vi "Sender UI.vi"(11 "error in (no error)":errorcluster) -> (15 "error out":errorcluster)   [LabVIEW 2023, in "Sender.lvclass"]
uses:
  Sender.lvclass
  Controls/Communication Mode.ctl
  Controls/Operation.ctl
  Controls/State Cluster.ctl
  Controls/Sender Data Cluster.ctl
  Communication/Communication.lvclass
  Controls/User Event Operation.ctl
  Downloads/Sample PC Template/Sample PC Template/Typedefs/Data.ctl
  Sender.lvclass/Sender.ctl
  Downloads/Sample PC Template/Sample PC Template/Sample PC Template.lvlib
panel:
  in  "Stop Data":bool
  in  "Transmission Type":T1
  in  "Data Type":string(combo)
  in  "Send":bool
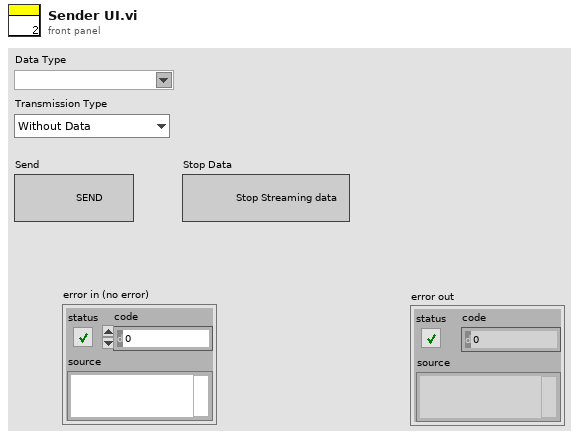
[diagram p1: front panel]
types:
  T1 = typedef "Communication Mode.ctl" = enum16{"Without Data", "With Data", "Stream Data"}
  T2 = typedef "User Event Operation.ctl" = enum16{"Obtain", "Generate", "Release"}
  T3 = typedef "Sender Data Cluster.ctl" = cluster{"user event out":refnum<user-event>, "Selected Data Type":string, "Receiver VI Reference":refnum<vi>, "Transmission Type":T1, "Start Time":dbl, "Stop Stream Data":bool, "Parent class object":refnum<class "Communication.lvclass">}
  T4 = typedef "State Cluster.ctl" = cluster{"State":string, "Data":variant}
  T5 = typedef "Operation.ctl" = enum16{"Create", "Enqueue", "Enqueue N", "Enstack", "Dequeue", "Flush", "Release"}
  T6 = typedef "Sample PC Template.lvlib/Data.ctl" = cluster{"State":string, "Data":variant}
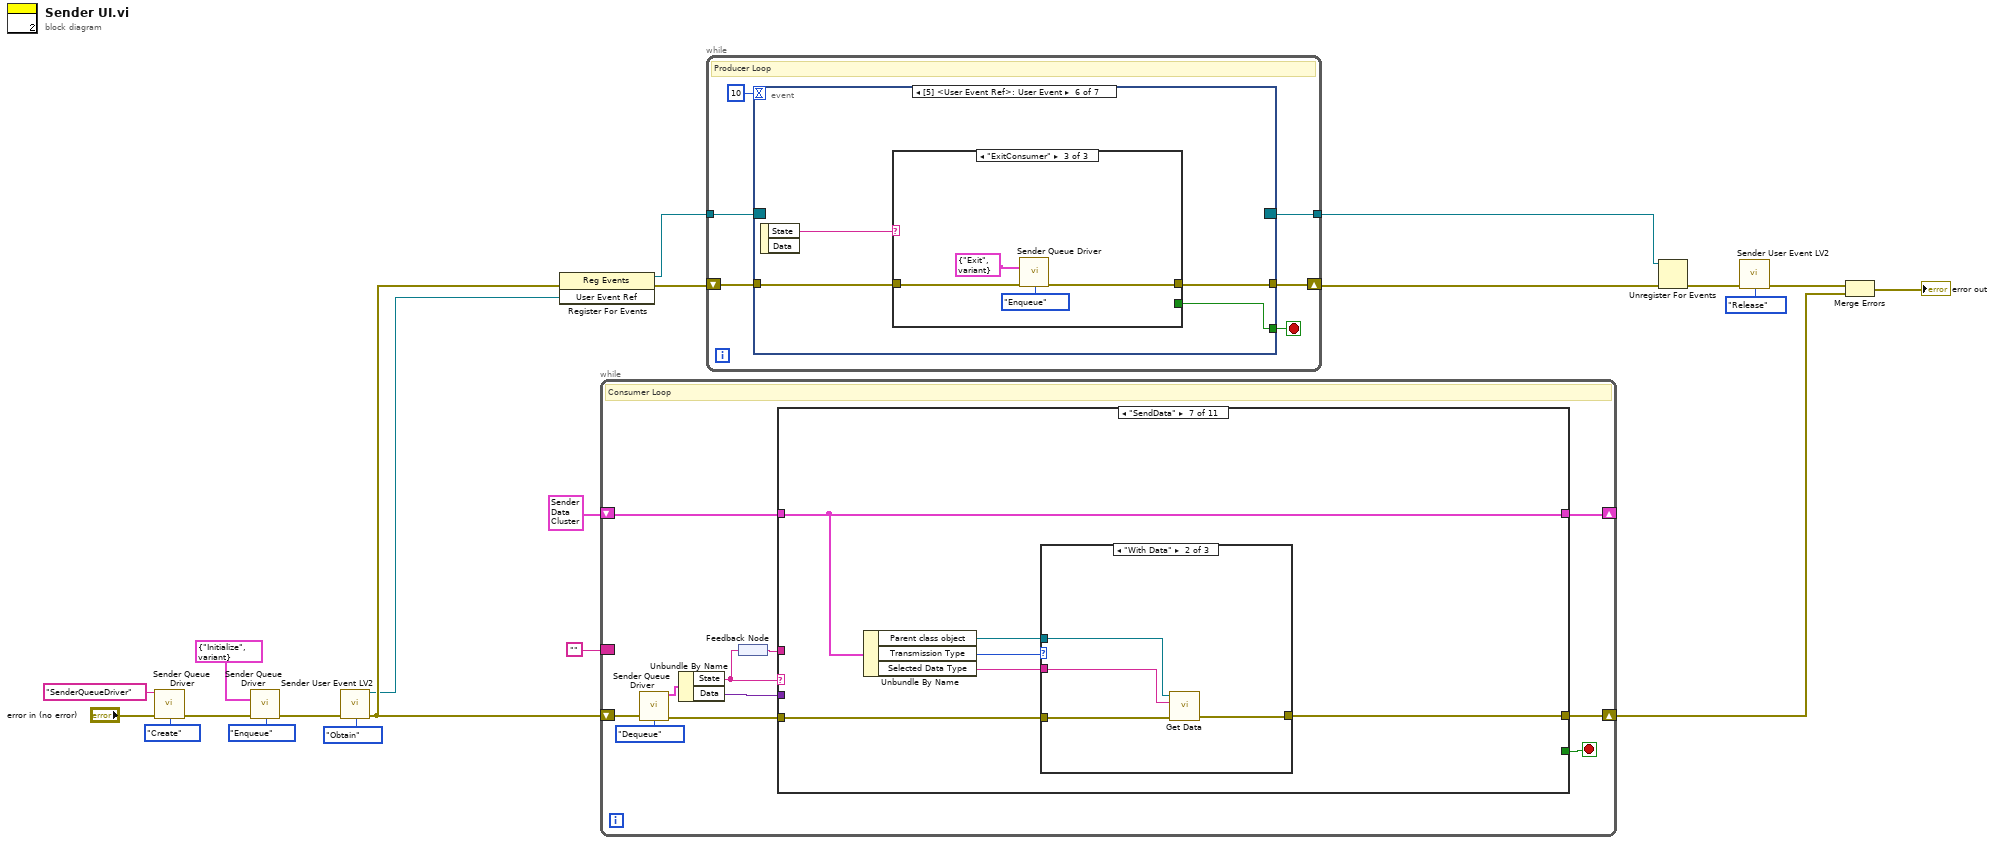
[diagram p0: block diagram]
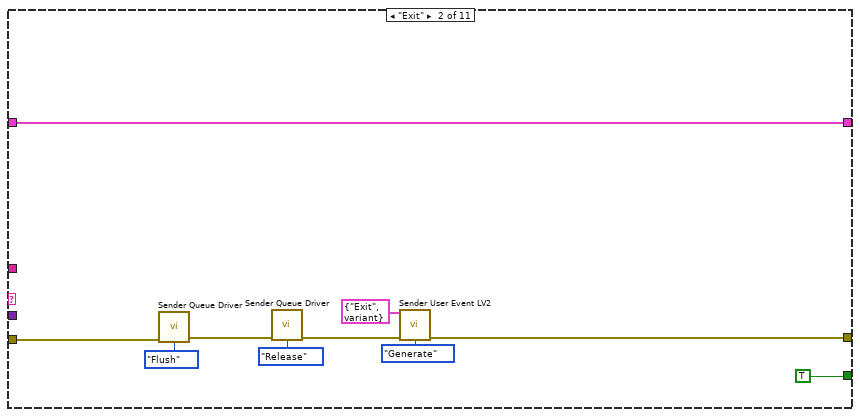
[diagram p3: hidden frame]
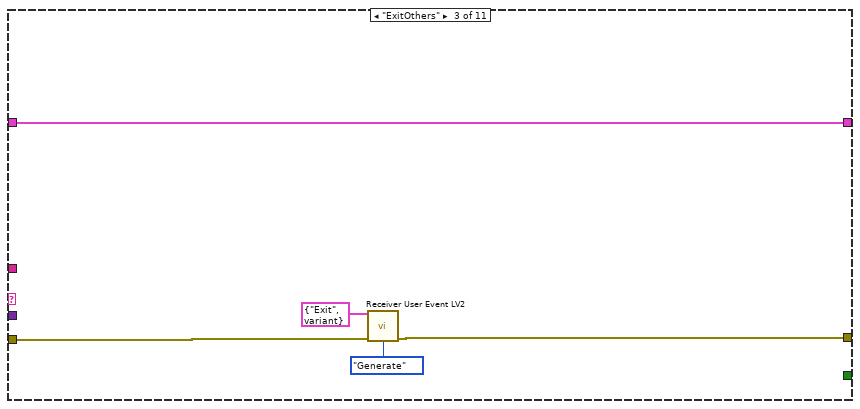
[diagram p4: hidden frame]
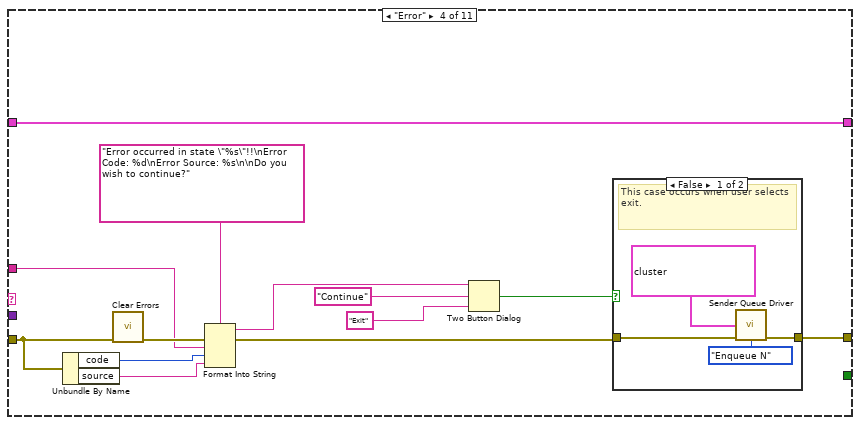
[diagram p5: hidden frame]
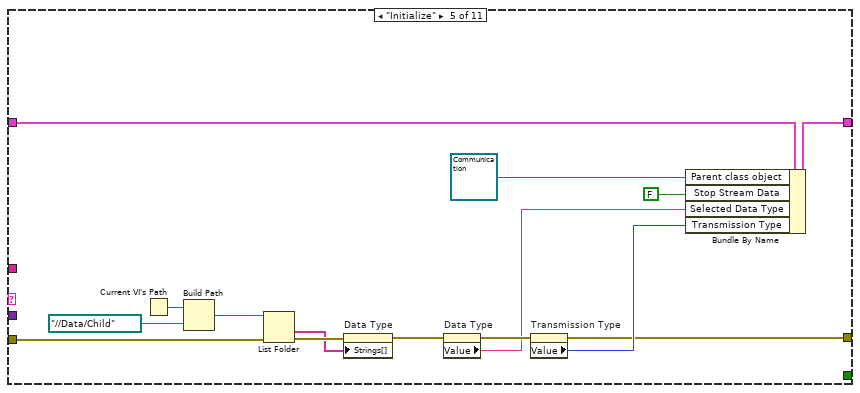
[diagram p7: hidden frame]
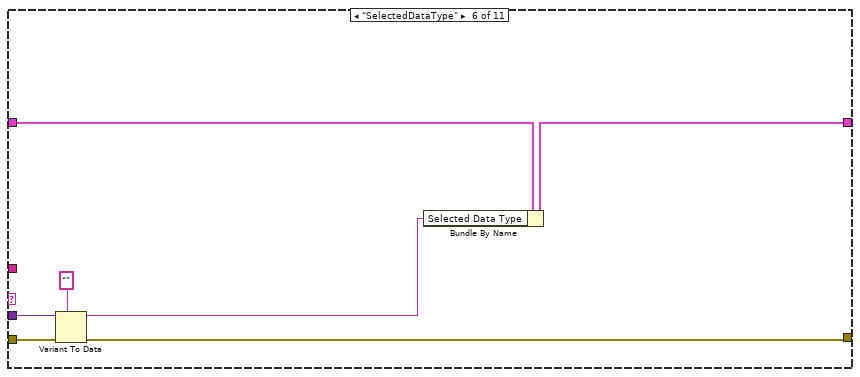
[diagram p8: hidden frame]
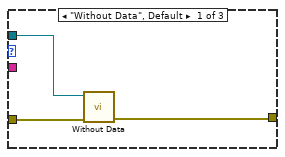
[diagram p9: hidden frame]
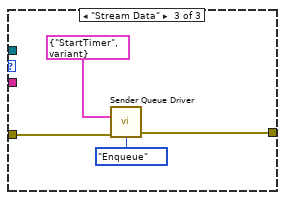
[diagram p10: hidden frame]
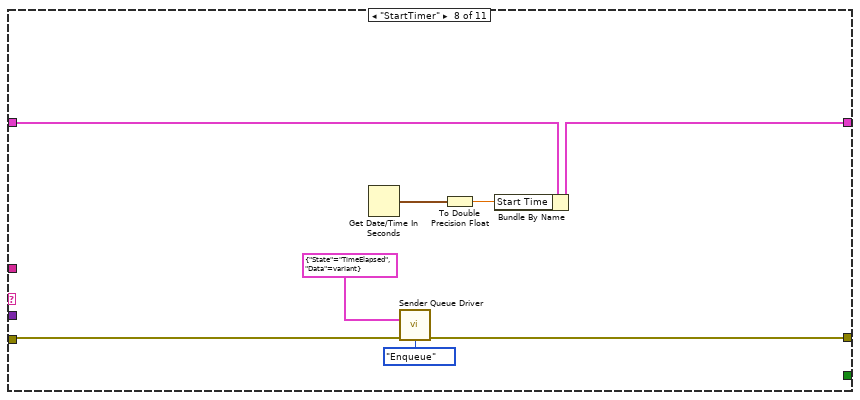
[diagram p11: hidden frame]
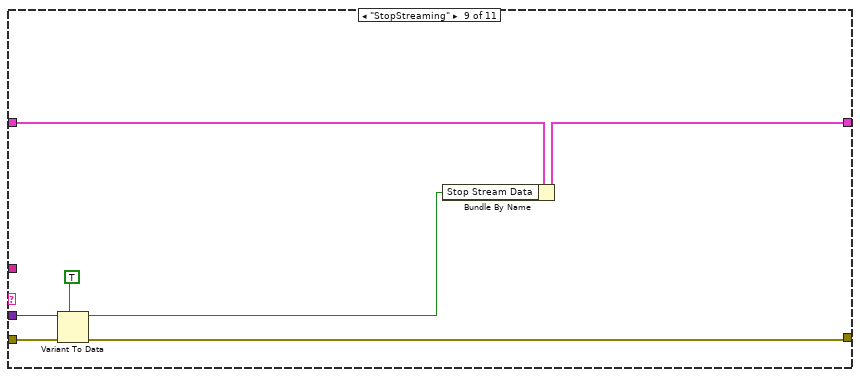
[diagram p12: hidden frame]
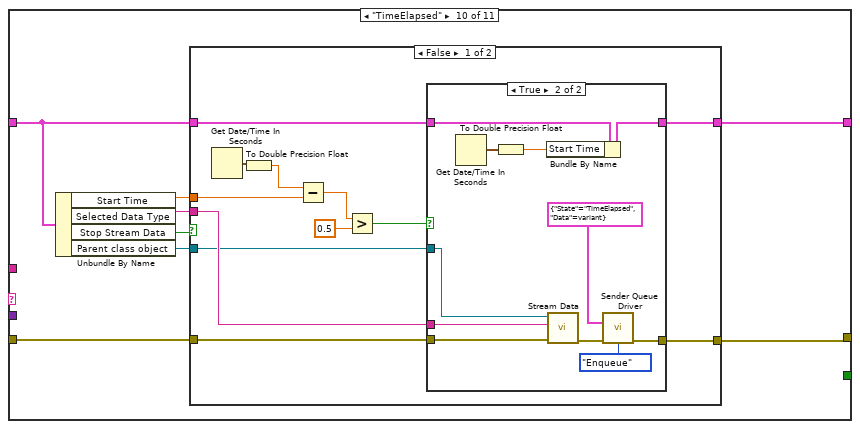
[diagram p13: hidden frame]
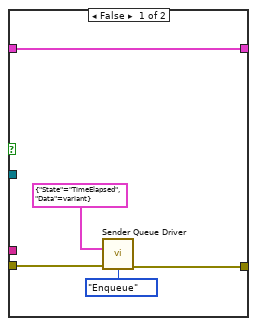
[diagram p14: hidden frame]
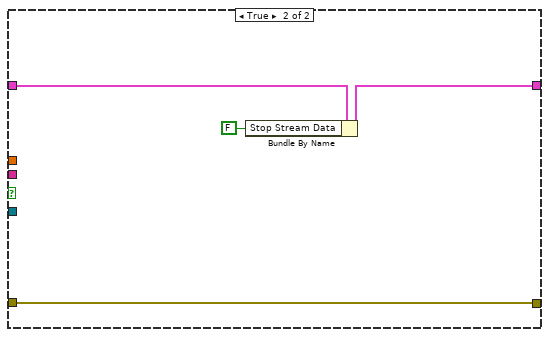
[diagram p15: hidden frame]
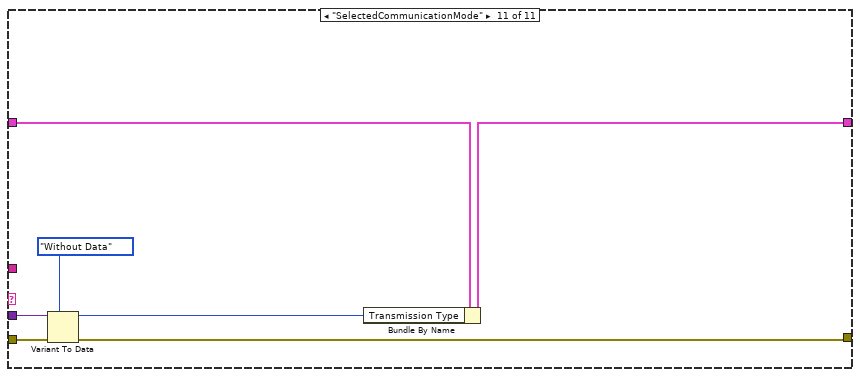
[diagram p16: hidden frame]
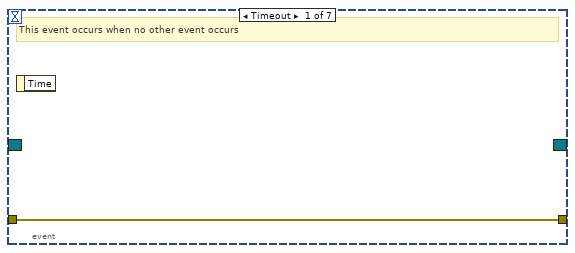
[diagram p17: hidden frame]
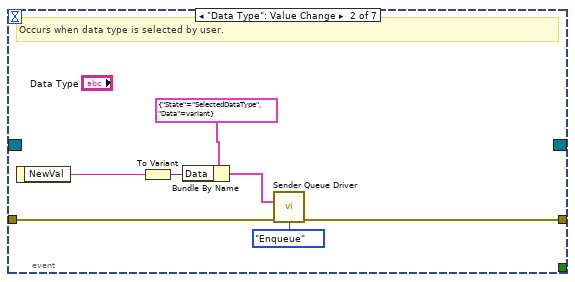
[diagram p18: hidden frame]
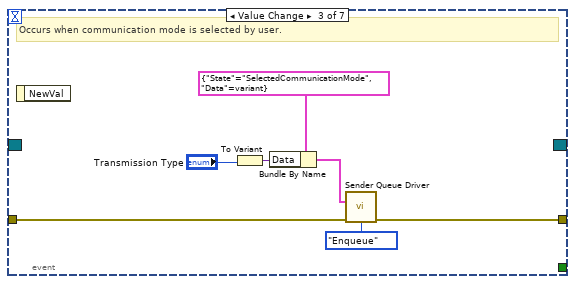
[diagram p19: hidden frame]
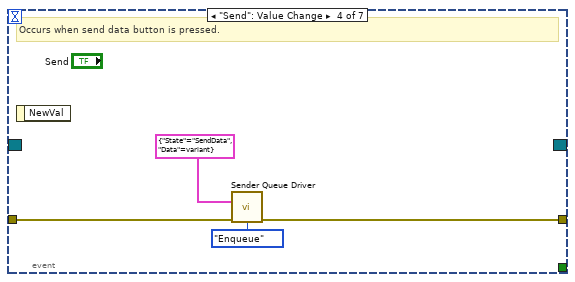
[diagram p20: hidden frame]
diagram:
  n1 = call "Sender Queue Driver.vi"("Queue Name"="SenderQueueDriver", "error in (no error)"="error in (no error)", "Operations"=Operation."Create") -> ("error out"=w19:errorcluster)  [unwired: 11 in, 1 out]
  n2 = call "Sender Queue Driver.vi"("State"=T4 {"State"="Initialize", "Data"=variant}, "error in (no error)"=w19, "Operations"=Operation."Enqueue") -> ("error out"=w7:errorcluster)  [unwired: 11 in, 1 out]
  n3 = call "Sender User Event LV2.vi"("Error In"=w7, "Operation"=User_Event_Operation."Obtain") -> ("User Event Ref"=w4:refnum<user-event>, "Error Out"=w6:errorcluster)  [unwired: 12 in]
  n4 = register-events(error in=w6, w4) -> (reference out=w13:refnum<event-registration>, error out=w14:errorcluster)  [unwired: 1 in]
  n5 = while {
    shift-right: [w25] -> w9
    shift-left: w6 -> [w31]
    border: "" -> [_]
    shift-right: [w22] -> _
    shift-left: T3 {"user event out"=refnum, "Selected Data Type"="", "Receiver VI Reference"=refnum, "Transmission Type"=enum."Without Data", "Start Time"=0.0, "Stop Stream Data"=FALSE, "Parent class object"=refnum} -> [w23]
    stop <- w24 stop-if-true
    # "Consumer Loop"
    n6 = call "Sender Queue Driver.vi"("error in (no error)"=w31, "Operations"=Operation."Dequeue") -> ("Dequeued Element"=w30:T4, "error out"=w28:errorcluster)  [unwired: 12 in]
    n7 = Unbundle By Name(w30) -> ("State"=w27:string, "Data"=w29:variant)
    n8 = feedback-in #1(w27) -> ()
    n9 = feedback #1() -> (w26:string)
    n10 = case shown="\"SendData\"" w27 {
      tunnel: w29 -> [_ _ _ _ _ w88 _ _ w118 _ w166]
      tunnel: w28 -> [w34 w43 w48 w55 w78 w89 w95 w110 w121 w128 w168]
      tunnel: w26 -> [_ _ _ w51 _ _ _ _ _ _ _]
      tunnel: [w34 w37 w47 w54 w69 w86 w94 w109 w120 w127 w167] -> w25
      tunnel: [_ TRUE _ _ _ _ _ _ _ _ _] -> w24
      tunnel: w23 -> [w33 w39 w49 w50 w82 w85 w93 w114 w117 w125 w164]
      tunnel: [w33 w39 w49 w50 w81 w84 w93 w113 w116 w124 w162] -> w22
      frame Default {
      }
      frame "Exit" {
        n11 = call "Sender Queue Driver.vi"("error in (no error)"=w43, "Operations"=Operation."Flush") -> ("error out"=w42:errorcluster)  [unwired: 12 in, 1 out]
        n12 = call "Sender Queue Driver.vi"("error in (no error)"=w42, "Operations"=Operation."Release") -> ("error out"=w38:errorcluster)  [unwired: 12 in, 1 out]
        n13 = call "Sender User Event LV2.vi"("Data"=T6 {"State"="Exit", "Data"=variant}, "Error In"=w38, "Operation"=User_Event_Operation."Generate") -> ("Error Out"=w37:errorcluster)  [unwired: 11 in, 1 out]
      }
      frame "ExitOthers" {
        n14 = call "Receiver User Event LV2.vi"("Data"=T6 {"State"="Exit", "Data"=variant}, "Error In"=w48, "Operation"=User_Event_Operation."Generate") -> ("Error Out"=w47:errorcluster)  [unwired: 11 in, 1 out]
      }
      frame "Error" {
        n15 = Unbundle By Name(w55) -> ("code"=w53:i32, "source"=w52:string)
        n16 = call <vilib>:"Clear Errors.vi"("error in (no error)"=w55) -> ("error out"=w62:errorcluster)  [unwired: 5 in, 1 out]
        n17 = Format Into String(format string="Error occurred in state \"%s\"!!\nError Code: %d\nError Source: %s\n\nDo you wish to continue?", error in=w62, w51, w53, w52) -> (resulting string=w60:string, error out=w57:errorcluster)  [unwired: 1 in]
        n18 = Two Button Dialog(message=w60, 1:"Exit" ("F button name (\"Cancel\")"), 2:"Continue" ("T button name (\"OK\")")) -> (T button?=w56:bool)
        n19 = case shown="False" w56 {
          tunnel: w57 -> [w64 w67]
          tunnel: [w66 w67] -> w54
          frame False {
            # "This case occurs when user selects exit."
            n20 = call "Sender Queue Driver.vi"("State []"=T4[] [{"State"="ExitOthers", "Data"=variant}, {"State"="Exit", "Data"=variant}], "error in (no error)"=w64, "Operations"=Operation."Enqueue N") -> ("error out"=w66:errorcluster)  [unwired: 11 in, 1 out]
          }
          frame True {
            # "This case occurs when user selects to continue."
          }
        }
      }
      frame "Initialize" {
        n21 = Current VI's Path() -> (path=w80:path)
        n22 = Build Path(base path=w80, name or relative path=path "../../Data/Child") -> (appended path=w77:path)
        n23 = List Folder(path=w77, error in=w78) -> (folder names=w75:string[], error out=w76:errorcluster)  [unwired: 2 in, 2 out]
        n24 = property on="Data Type" class="CmbBox"(error in=w76, "Strings[]"=w75) -> (error out=w73:errorcluster)  [unwired: 1 in, 1 out]
        n25 = property on="Data Type" class="CmbBox"(error in=w73) -> (error out=w72:errorcluster, "Value"=w70:string)  [unwired: 1 in, 1 out]
        n26 = property on="Transmission Type" class="Enum (strict)"(error in=w72) -> (error out=w69:errorcluster, "Value"=w71:T1)  [unwired: 1 in, 1 out]
        n27 = Bundle By Name(cluster=w82, "Parent class object"=refnum<class "Communication.lvclass"> refnum ("Communication.lvclass"), "Stop Stream Data"=FALSE, "Selected Data Type"=w70, "Transmission Type"=w71) -> (w81:T3)
      }
      frame "SelectedDataType" {
        n28 = Variant To Data(error in=w89, type="", Variant=w88) -> (data=w83:string, error out=w86:errorcluster)
        n29 = Bundle By Name(cluster=w85, "Selected Data Type"=w83) -> (w84:T3)
      }
      frame "SendData" {
        n30 = Unbundle By Name(w93) -> ("Parent class object"=w90:refnum<class "Communication.lvclass">, "Transmission Type"=w92:T1, "Selected Data Type"=w91:string)
        n31 = case shown="\"With Data\"" w92 {
          tunnel: w95 -> [w98 w102 w106]
          tunnel: [w96 w101 w105] -> w94
          tunnel: w91 -> [_ w100 _]
          tunnel: w90 -> [w97 w99 _]
          frame "Without Data", Default {
            n32 = call "Without Data.vi"("error in (no error)"=w98, "Communication in"=w97) -> ("error out"=w96:errorcluster)  [unwired: 8 in, 1 out]
          }
          frame "With Data" {
            n33 = call "Get Data.vi"("error in (no error)"=w102, "Data Type"=w100, "Communication in"=w99) -> ("error out"=w101:errorcluster)  [unwired: 7 in, 1 out]
          }
          frame "Stream Data" {
            n34 = call "Sender Queue Driver.vi"("State"=T4 {"State"="StartTimer", "Data"=variant}, "error in (no error)"=w106, "Operations"=Operation."Enqueue") -> ("error out"=w105:errorcluster)  [unwired: 11 in, 1 out]
          }
        }
      }
      frame "StartTimer" {
        n35 = Get Date/Time In Seconds() -> (seconds since 1Jan1904=w111:timestamp)
        n36 = call "Sender Queue Driver.vi"("State"=T4 {"State"="TimeElapsed", "Data"=variant}, "error in (no error)"=w110, "Operations"=Operation."Enqueue") -> ("error out"=w109:errorcluster)  [unwired: 11 in, 1 out]
        n37 = To Double Precision Float(number=w111) -> (double precision float=w112:dbl)
        n38 = Bundle By Name(cluster=w114, "Start Time"=w112) -> (w113:T3)
      }
      frame "StopStreaming" {
        n39 = Variant To Data(error in=w121, type=TRUE, Variant=w118) -> (data=w115:bool, error out=w120:errorcluster)
        n40 = Bundle By Name(cluster=w117, "Stop Stream Data"=w115) -> (w116:T3)
      }
      frame "TimeElapsed" {
        n41 = Unbundle By Name(w125) -> ("Start Time"=w129:dbl, "Selected Data Type"=w126:string, "Stop Stream Data"=w123:bool, "Parent class object"=w122:refnum<class "Communication.lvclass">)
        n42 = case shown="False" w123 {
          tunnel: w129 -> [w131 _]
          tunnel: w128 -> [w138 w161]
          tunnel: [w137 w161] -> w127
          tunnel: w126 -> [w135 _]
          tunnel: w125 -> [w134 w160]
          tunnel: [w133 w158] -> w124
          tunnel: w122 -> [w130 _]
          frame False {
            n43 = Get Date/Time In Seconds() -> (seconds since 1Jan1904=w141:timestamp)
            n44 = To Double Precision Float(number=w141) -> (double precision float=w132:dbl)
            n45 = Subtract(x=w132, y=w131) -> (x-y=w140:dbl)
            n46 = Greater?(x=w140, y=0.5) -> (0:w136:bool)
            n47 = case shown="True" w136 {
              tunnel: w138 -> [w146 w157]
              tunnel: [w145 w150] -> w137
              tunnel: w135 -> [_ w156]
              tunnel: w134 -> [w142 w155]
              tunnel: [w142 w154] -> w133
              tunnel: w130 -> [_ w147]
              frame False {
                n48 = call "Sender Queue Driver.vi"("State"=T4 {"State"="TimeElapsed", "Data"=variant}, "error in (no error)"=w146, "Operations"=Operation."Enqueue") -> ("error out"=w145:errorcluster)  [unwired: 11 in, 1 out]
              }
              frame True {
                n49 = Get Date/Time In Seconds() -> (seconds since 1Jan1904=w153:timestamp)
                n50 = To Double Precision Float(number=w153) -> (double precision float=w152:dbl)
                n51 = Bundle By Name(cluster=w155, "Start Time"=w152) -> (w154:T3)
                n52 = call "Stream Data.vi"("error in (no error)"=w157, "Data Type"=w156, "Communication in"=w147) -> ("error out"=w151:errorcluster)  [unwired: 7 in, 1 out]
                n53 = call "Sender Queue Driver.vi"("State"=T4 {"State"="TimeElapsed", "Data"=variant}, "error in (no error)"=w151, "Operations"=Operation."Enqueue") -> ("error out"=w150:errorcluster)  [unwired: 11 in, 1 out]
              }
            }
          }
          frame True {
            n54 = Bundle By Name(cluster=w160, "Stop Stream Data"=FALSE) -> (w158:T3)
          }
        }
      }
      frame "SelectedCommunicationMode" {
        n55 = Variant To Data(error in=w168, type=Communication_Mode."Without Data" ("Communication Mode"), Variant=w166) -> (data=w163:T1, error out=w167:errorcluster)
        n56 = Bundle By Name(cluster=w164, "Transmission Type"=w163) -> (w162:T3)
      }
    }
  }
  n57 = while {
    shift-right: [w171] -> w11
    shift-left: w14 -> [w172]
    tunnel: w13 -> [w173]
    tunnel: [w169] -> w10
    stop <- w170 stop-if-true
    # "Producer Loop"
    n58 = event shown="[5] <User Event Ref>: User Event" {
      selector: w173 -> [_ _ _ _ _ _ _]
      dyn-events: [_ _ _ _ _ _ _] -> w169
      timeout: 10 -> [_ _ _ _ _ _ _]
      tunnel: w172 -> [w175 w182 w189 w193 w200 w203 w215]
      tunnel: [w175 w181 w188 w192 w199 w201 w214] -> w171
      tunnel: [_ _ _ _ _ w202 _] -> w170
      event Timeout {
        # "This event occurs when no other event occurs"
        n59 = event-data() -> ()  [unwired: 1 in, 1 out]
      }
      event "Data Type": Value Change {
        # "Occurs when data type is selected by user."
        n60 = event-data() -> ("NewVal"=w177:string)  [unwired: 1 in]
        n61 = To Variant(anything=w177) -> (Variant=w178:variant)
        n62 = Bundle By Name(cluster=T4 {"State"="SelectedDataType", "Data"=variant} ("State"), "Data"=w178) -> (w176:T4)
        n63 = call "Sender Queue Driver.vi"("State"=w176, "error in (no error)"=w182, "Operations"=Operation."Enqueue") -> ("error out"=w181:errorcluster)  [unwired: 11 in, 1 out]
      }
      event Value Change {
        # "Occurs when communication mode is selected by user."
        n64 = event-data() -> ()  [unwired: 1 in, 1 out]
        n65 = To Variant(anything="Transmission Type") -> (Variant=w184:variant)
        n66 = Bundle By Name(cluster=T4 {"State"="SelectedCommunicationMode", "Data"=variant} ("State"), "Data"=w184) -> (w183:T4)
        n67 = call "Sender Queue Driver.vi"("State"=w183, "error in (no error)"=w189, "Operations"=Operation."Enqueue") -> ("error out"=w188:errorcluster)  [unwired: 11 in, 1 out]
      }
      event "Send": Value Change {
        # "Occurs when send data button is pressed."
        n68 = event-data() -> ()  [unwired: 1 in, 1 out]
        n69 = call "Sender Queue Driver.vi"("State"=T4 {"State"="SendData", "Data"=variant}, "error in (no error)"=w193, "Operations"=Operation."Enqueue") -> ("error out"=w192:errorcluster)  [unwired: 11 in, 1 out]
      }
      event "Stop Data": Value Change {
        # "Occurs when stop streaming data is pressed."
        n70 = event-data() -> ()  [unwired: 1 in, 1 out]
        n71 = To Variant(anything=TRUE) -> (Variant=w196:variant)
        n72 = Bundle By Name(cluster=T4 {"State"="StopStreaming", "Data"=variant} ("State"), "Data"=w196) -> (w194:T4)
        n73 = call "Sender Queue Driver.vi"("State"=w194, "error in (no error)"=w200, "Operations"=Operation."Enqueue") -> ("error out"=w199:errorcluster)  [unwired: 11 in, 1 out]
      }
      event User Event {
        n74 = event-data() -> ("State"=w204:string)  [unwired: 1 in, 1 out]
        n75 = case shown="\"ExitConsumer\"" w204 {
          tunnel: w203 -> [w205 w206 w211]
          tunnel: [_ TRUE ("Discard?") _] -> w202
          tunnel: [w205 w206 w210] -> w201
          frame Default {
          }
          frame "Exit" {
          }
          frame "ExitConsumer" {
            n76 = call "Sender Queue Driver.vi"("State"=T4 {"State"="Exit", "Data"=variant}, "error in (no error)"=w211, "Operations"=Operation."Enqueue") -> ("error out"=w210:errorcluster)  [unwired: 11 in, 1 out]
          }
        }
      }
      event Panel Close? {
        # "Occurs when panel close is pressed"
        n77 = event-data() -> ()  [unwired: 1 in, 1 out]
        n78 = call "Sender Queue Driver.vi"("State []"=T4[] [{"State"="ExitOthers", "Data"=variant}, {"State"="Exit", "Data"=variant}], "error in (no error)"=w215, "Operations"=Operation."Enqueue N") -> ("error out"=w214:errorcluster)  [unwired: 11 in, 1 out]
        n79 = event-data("Discard?"=TRUE) -> ()  [unwired: 1 in, 1 out]
      }
    }
  }
  n80 = Unregister For Events(event registration refnum=w10, error in=w11) -> (error out=w3:errorcluster)
  n81 = call "Sender User Event LV2.vi"("Error In"=w3, "Operation"=User_Event_Operation."Release") -> ("Error Out"=w2:errorcluster)  [unwired: 12 in, 1 out]
  n82 = Merge Errors(w2, w9) -> (→"error out":errorcluster)
